vi "enqueue_data.vi"(0 "Active Analog Data In":T1[](array[typedef]), 5 "Label indicies In":i32[](array[numeric]), 7 "timestamp":dbl[](array[numeric]), 9 "# of Samples":u32, 11 "error in":errorcluster, 12 "data Queue":refnum<queue>, 13 "Record dP Data":refnum<vi>, 14 "dP Recording Progress":refnum<vi>) -> (15 "error out":errorcluster)   [LabVIEW 2017]
uses:
  Input Channel Lists/analog_data.ctl
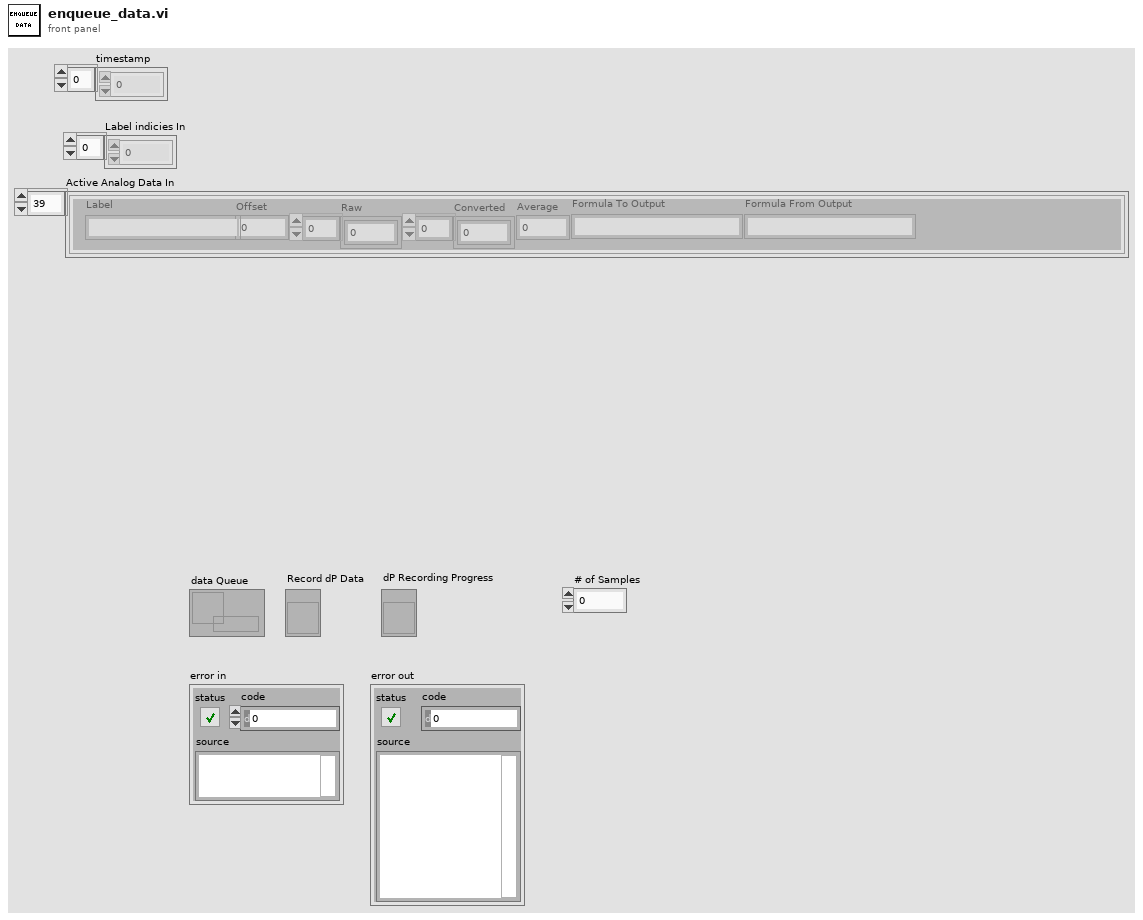
[diagram p1: front panel]
types:
  T1 = typedef "analog_data.ctl" = cluster{"Label":string, "Offset":dbl, "Raw":dbl[], "Converted":dbl[], "Average":dbl, "Formula To Output":string, "Formula From Output":string}
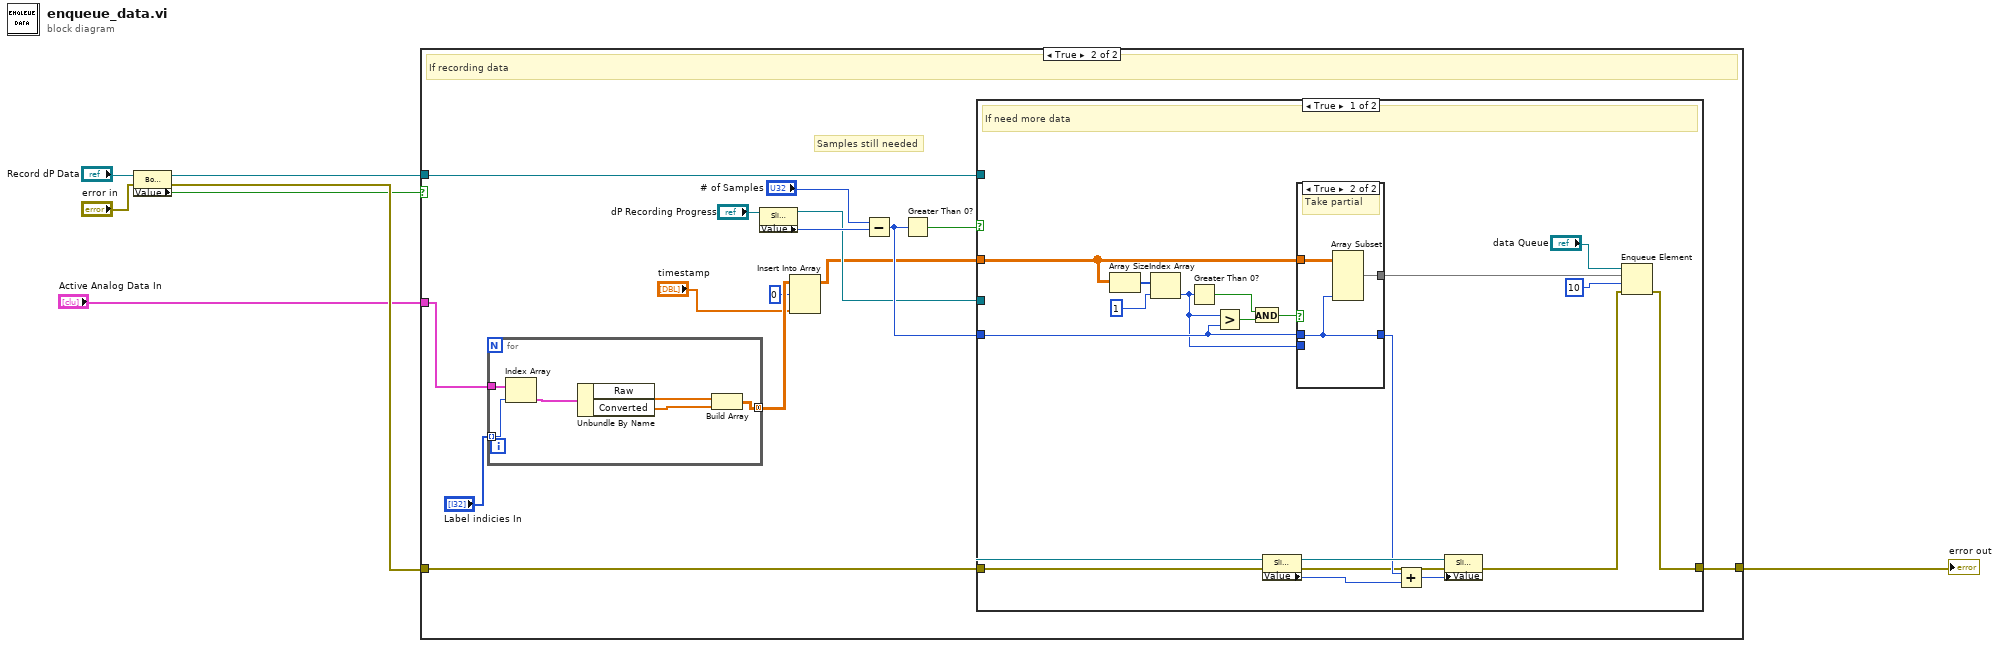
[diagram p0: block diagram]
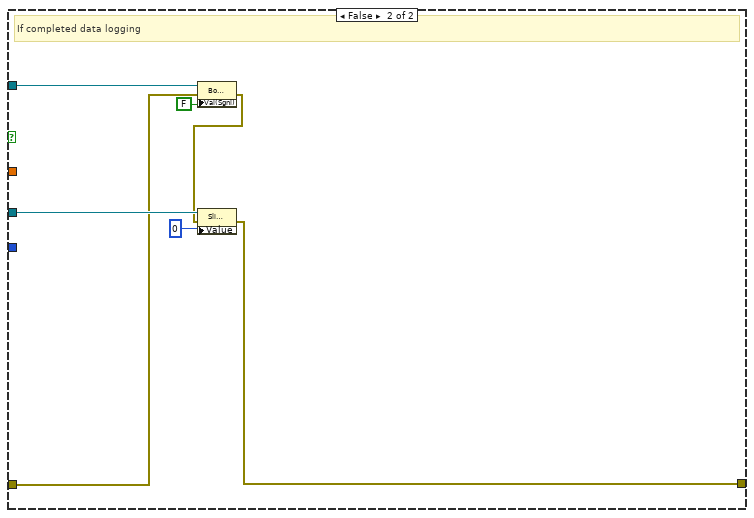
[diagram p4: hidden frame]
diagram:
  n1 = property class="Bool (strict)"(reference="Record dP Data", error in="error in") -> (reference out=w6:refnum<vi>, error out=w4:errorcluster, "Value"=w2:bool)
  n2 = case shown="True" w2 {
    tunnel: w6 -> [_ w17]
    tunnel: [w8 w16] -> w5
    tunnel: w4 -> [w8 w15]
    tunnel: "Active Analog Data In" -> [_ w13]
    frame False {
      # "If not recording data, do nothing"
    }
    frame True {
      # "Samples still needed"
      # "If recording data"
      n3 = for {
        tunnel: [w29] -> w12 mode=concatenating
        tunnel: w13 -> [w26]
        tunnel: "Label indicies In" -> [w25] mode=indexing
        n4 = Index Array(array=w26, index=w25) -> (element=w24:T1)
        n5 = Unbundle By Name(w24) -> ("Raw"=w28:dbl[], "Converted"=w27:dbl[])
        n6 = Build Array(w28, w27) -> (w29:dbl[][])
      }
      n7 = property class="Slide (strict)"(reference="dP Recording Progress") -> (reference out=w18:refnum<vi>, "Value"=w22:u32)  [unwired: 1 in, 1 out]
      n8 = Insert Into Array(array=w12, index (row)=0, new element="timestamp") -> (w10:dbl[][])  [unwired: 1 in]
      n9 = Subtract(x="# of Samples", y=w22) -> (x-y=w19:u32)
      n10 = Greater Than 0?(x=w19) -> (x > 0?=w20:bool)
      n11 = case shown="True" w20 {
        tunnel: w19 -> [w47 _]
        tunnel: w18 -> [w40 w59]
        tunnel: w17 -> [_ w58]
        tunnel: w10 -> [w35 _]
        tunnel: [w30 w56] -> w16
        tunnel: w15 -> [w32 w55]
        frame True {
          # "If need more data"
          n12 = Array Size(array=w35) -> (size(s)=w49:i32[])
          n13 = Index Array(array=w49, index=1) -> (element=w43:i32)
          n14 = Greater Than 0?(x=w43) -> (x > 0?=w46:bool)
          n15 = Greater?(x=w43, y=w47) -> (0:w45:bool)
          n16 = And(x=w46, y=w45) -> (x .and. y?=w44:bool)
          n17 = property class="Slide (strict)"(reference=w40, error in=w32) -> (reference out=w38:refnum<vi>, error out=w33:errorcluster, "Value"=w39:u32)
          n18 = case shown="True" w44 {
            tunnel: w35 -> [w51 w54]
            tunnel: w47 -> [_ w52]
            tunnel: [w51 w53] -> w34
            tunnel: [w50 w52] -> w36
            tunnel: w43 -> [w50 _]
            frame False {
              # "Take all"
            }
            frame True {
              # "Take partial"
              n19 = Array Subset(array=w54, length (col)=w52) -> (w53:dbl[][])  [unwired: 3 in]
            }
          }
          n20 = Add(x=w36, y=w39) -> (x+y=w37:u32)
          n21 = property class="Slide (strict)"(reference=w38, error in=w33, "Value"=w37) -> (error out=w31:errorcluster)  [unwired: 1 out]
          n22 = Enqueue Element(queue="data Queue", element=w34, timeout in ms (-1)=10, error in (no error)=w31) -> (error out=w30:errorcluster)  [unwired: 2 out]
        }
        frame False {
          # "If completed data logging"
          n23 = property class="Bool (strict)"(reference=w58, error in=w55, "Val(Sgnl)"=FALSE ("Value (Signaling)")) -> (error out=w57:errorcluster)  [unwired: 1 out]
          n24 = property class="Slide (strict)"(reference=w59, error in=w57, "Value"=u32 0 ("dP Recording Progress")) -> (error out=w56:errorcluster)  [unwired: 1 out]
        }
      }
    }
  }
  "error out" <- w5
